vi "Update_Error_Table_Data.vi"(0 "Error_Data_In":T1, 2 "Table_Reference":refnum<vi>, 5 "Error_Message":string, 11 "Error_In":errorcluster) -> (4 "Error_Data_Out":T1, 6 "Error_Table_Data":string[][](array[string]), 15 "Error_Out":errorcluster)   [LabVIEW 2021]
doc: "Used to update the error table."
uses:
  Controls/Error_Data.ctl
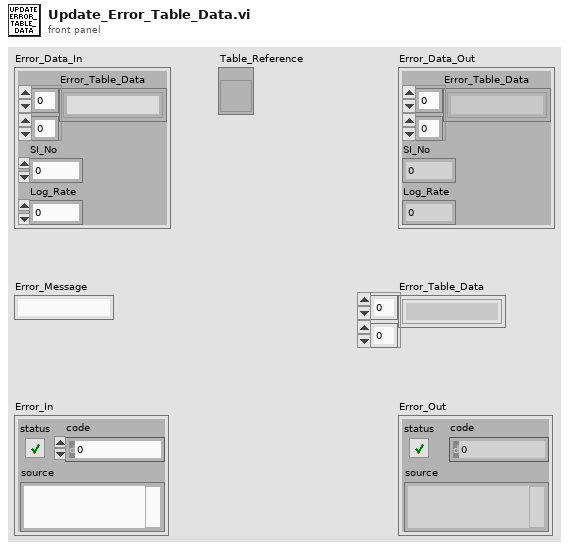
[diagram p1: front panel]
types:
  T1 = typedef "Error_Data.ctl" = cluster{"Error_Table_Data":string[][], "SI_No":i32, "Log_Rate":u32}
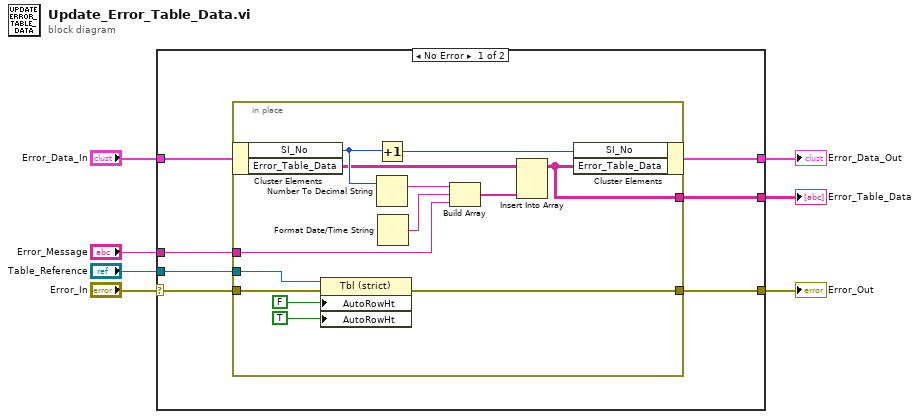
[diagram p0: block diagram]
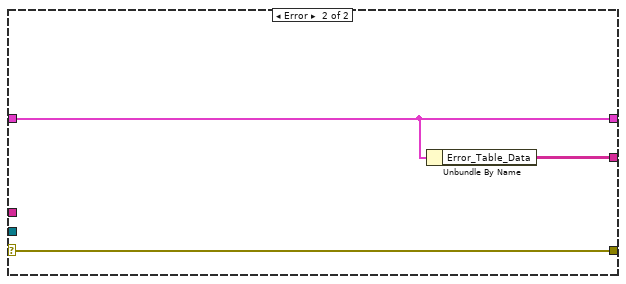
[diagram p2: hidden frame]
diagram:
  n1 = case shown="No Error" "Error_In" {
    selector: "Error_In" -> [w8 w30]
    tunnel: [w14 w28] -> w7
    tunnel: "Error_Data_In" -> [w13 w29]
    tunnel: "Error_Message" -> [w12 _]
    tunnel: [w11 w30] -> w4
    tunnel: [w10 w29] -> w3
    tunnel: "Table_Reference" -> [w9 _]
    frame No Error {
      n2 = in-place {
        in-place-border: [w17] -> w11
        in-place-border: w8 -> [w18]
        in-place-border: w12 -> [w19]
        in-place-border: [w16] -> w14
        in-place-border: w9 -> [w15]
        n3 = in-place-cluster #1(w13) -> ("SI_No"=w25:i32, "Error_Table_Data"=w24:string[][])
        n4 = property on="Property Node" class="Tbl (strict)"(reference=w15, error in=w18, "AutoRowHt"=FALSE ("Autosizing Row Height"), "AutoRowHt"=TRUE ("Autosizing Row Height")) -> (error out=w17:errorcluster)  [unwired: 1 out]
        n5 = Increment(x=w25) -> (x+1=w23:i32)
        n6 = Number To Decimal String(number=w25) -> (decimal integer string=w27:string)  [unwired: 1 in]
        n7 = Format Date/Time String() -> (date/time string=w26:string)  [unwired: 3 in]
        n8 = Build Array(w27, w26, w19) -> (w20:string[])
        n9 = Insert Into Array(array=w24, new element=w20) -> (w16:string[][])  [unwired: 2 in]
        n10 = in-place-cluster #1("SI_No"=w23, "Error_Table_Data"=w16) -> (w10:T1)
      }
    }
    frame Error {
      n11 = Unbundle By Name(w29) -> ("Error_Table_Data"=w28:string[][])
    }
  }
  "Error_Table_Data" <- w7
  "Error_Out" <- w4
  "Error_Data_Out" <- w3
